vi "Parse lvproj with Virtual Folder1.vi"(11 "Test Case In":refnum<class "Parsing XML.lvclass">) -> (0 "error out":errorcluster, 3 "Test Case Out":refnum<class "Parsing XML.lvclass">)   [LabVIEW 2020, in "Parsing XML.lvclass"]
uses:
  Parsing XML.lvclass
  4993e8ee-a06a-463a-9684-69129f64d5ce.vi
  source/VI Properties Editor.lvlib
panel:
  out "Array":string[](array[string])
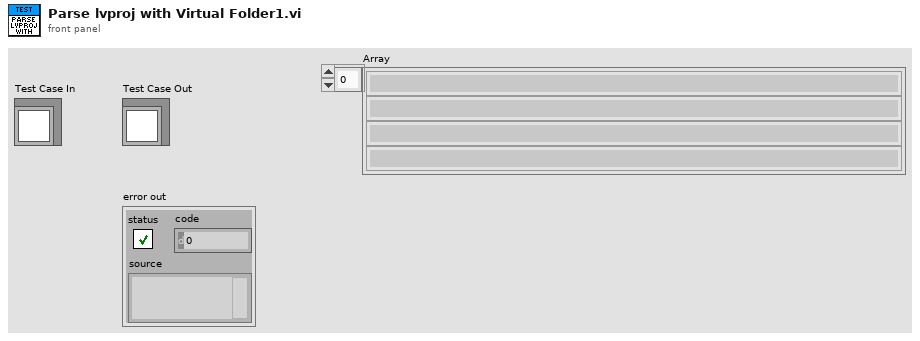
[diagram p1: front panel]
types:
  T1 = typedef "VI Properties Editor.lvlib/VI Data.ctl" = cluster{"VI":T2, "Ctl Properties":T4[], "Hierarchy":string}
  T2 = typedef "VI Properties Editor.lvlib/VI Properties.ctl" = cluster{"Name":string, "Path":path, "Type":enum32{"invalid VI type", "Standard VI", "Control VI", "Global VI", "Polymorphic VI", "Configuration VI", "SubSystem", "Facade VI", "Method VI", "Statechart Diagram VI"}, "Window Title":string, "Description":string, "Help Path":path, "Help Tag":string, "Help Web URL":string, "Use Web URL?":bool, "Custom Title?":bool, "Allow Debugging?":bool, "Reentrant?":bool, "Inlined?":bool, "Reentrancy Type":enum16{"Share clones between instances", "Preallocate clone for each instance"}, "Priority":enum32{"invalid priority", "background priority", "normal priority", "above normal priority", "high priority", "time critical priority", "subroutine"}, "Preferred Exec System":enum32{"invalid execution system", "user interface", "standard", "instrument i/o", "data acquisition", "other 1", "other 2", "same as caller"}, "Auto Error Handling?":bool, "Run When Opened?":bool, "Suspend When Called?":bool, "Conpane Img":T3}
  T3 = typedef "imagedata.ctl" = cluster{"image type":i32, "image depth":i32, "image":u8[], "mask":u8[], "colors":u32[], "Rectangle":cluster{"left":i16, "top":i16, "right":i16, "bottom":i16}}
  T4 = typedef "VI Properties Editor.lvlib/Control Properties.ctl" = cluster{"UID":i32, "Name":string, "Caption":string, "Description":string, "Tip Strip":string, "Is Indicator?":bool, "Is on ConPane?":bool}
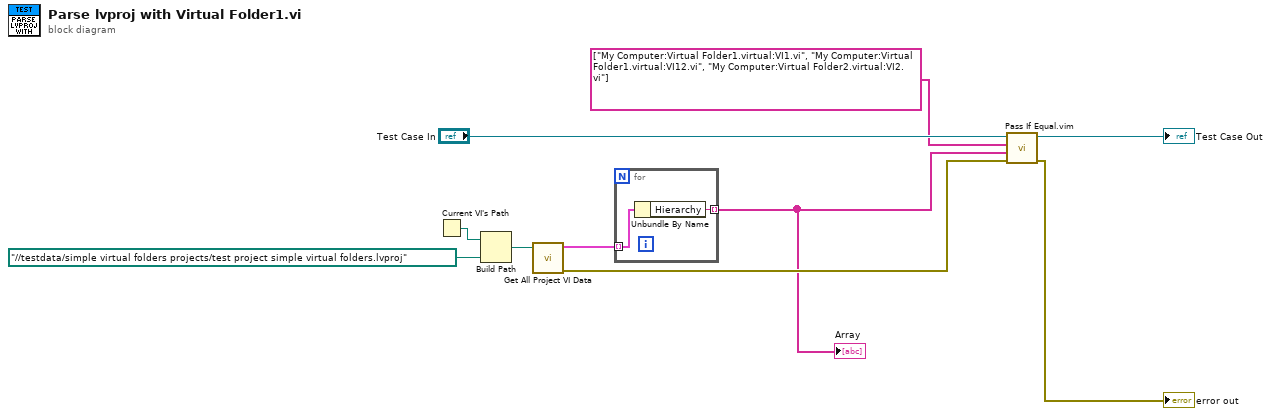
[diagram p0: block diagram]
diagram:
  n1 = Current VI's Path() -> (path=w7:path)
  n2 = Build Path(base path=w7, name or relative path=path "../../testdata/simple virtual folders projects/test project simple virtual folders.lvproj") -> (appended path=w2:path)
  n3 = call "Get All Project VI Data.vi"("Lvproj Path"=w2) -> ("error out"=w6:errorcluster, "VI Data"=w5:T1[])  [unwired: 9 in]
  n4 = for {
    tunnel: w5 -> [w12] mode=indexing
    tunnel: [w11] -> w4 mode=indexing
    n5 = Unbundle By Name(w12) -> ("Hierarchy"=w11:string)
  }
  "Array" <- w4
  n6 = call "Pass If Equal.vim"("error in (no error)"=w6, "Actual"=w4, "Expected"=string[] ["My Computer:Virtual Folder1.virtual:VI1.vi", "My Computer:Virtual Folder1.virtual:VI12.vi", "My Computer:Virtual Folder2.virtual:VI2.vi"] ("Array"), "LUnit Test Case In"="Test Case In") -> ("error out"=→"error out":errorcluster, "LUnit Test Case Out"=→"Test Case Out":refnum<class "Parsing XML.lvclass">)  [unwired: 6 in]
